vi "GetMotorCMD.vi"(11 "Notifiers":T1) -> (0 "PanCameraCMD":i32, 1 "LeftRudderCMD":i32, 2 "StarboardMotorCMD":i32, 3 "PCStatusCMD":i32, 4 "RightRudderCMD":i32, 5 "PortMotorCMD":i32)   [LabVIEW 2012]
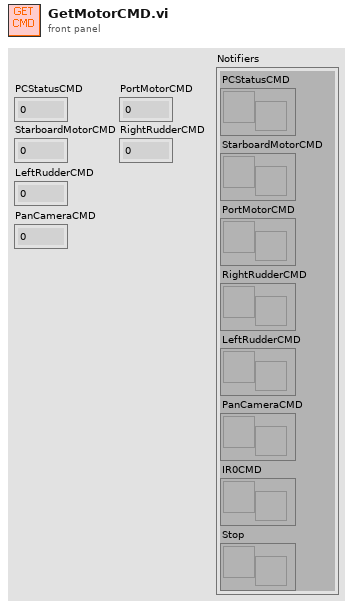
[diagram p1: front panel]
types:
  T1 = cluster{"PCStatusCMD":refnum<notifier>, "StarboardMotorCMD":refnum<notifier>, "PortMotorCMD":refnum<notifier>, "RightRudderCMD":refnum<notifier>, "LeftRudderCMD":refnum<notifier>, "PanCameraCMD":refnum<notifier>, "IR0CMD":refnum<notifier>, "Stop":refnum<notifier>}
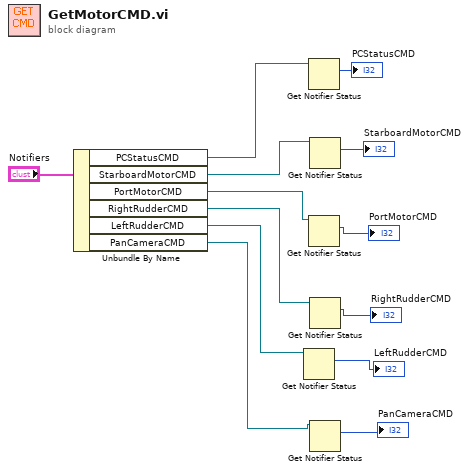
[diagram p0: block diagram]
diagram:
  n1 = Unbundle By Name("Notifiers") -> ("PCStatusCMD"=w13:refnum<notifier>, "StarboardMotorCMD"=w12:refnum<notifier>, "PortMotorCMD"=w11:refnum<notifier>, "RightRudderCMD"=w10:refnum<notifier>, "LeftRudderCMD"=w9:refnum<notifier>, "PanCameraCMD"=w8:refnum<notifier>)
  n2 = Get Notifier Status(notifier=w9) -> (current notification=→"LeftRudderCMD":i32)  [unwired: 1 in, 4 out]
  n3 = Get Notifier Status(notifier=w13) -> (current notification=→"PCStatusCMD":i32)  [unwired: 1 in, 4 out]
  n4 = Get Notifier Status(notifier=w11) -> (current notification=→"PortMotorCMD":i32)  [unwired: 1 in, 4 out]
  n5 = Get Notifier Status(notifier=w12) -> (current notification=→"StarboardMotorCMD":i32)  [unwired: 1 in, 4 out]
  n6 = Get Notifier Status(notifier=w10) -> (current notification=→"RightRudderCMD":i32)  [unwired: 1 in, 4 out]
  n7 = Get Notifier Status(notifier=w8) -> (current notification=→"PanCameraCMD":i32)  [unwired: 1 in, 4 out]
